vi "Main.vi"   [LabVIEW 2021]
uses:
  Hello World Event/Hello World Event/Hello World Event.lvclass
  C:/Program Files/National Instruments/LabVIEW 2021/vi.lib/Nathan Davis/jettl/jettl/Event/Event.lvclass
  <vilib>/Nathan Davis/jettl/jettl/jettl.lvlib
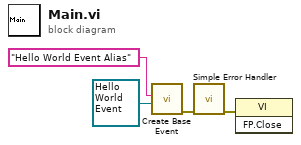
[diagram p0: block diagram]
diagram:
  n1 = call <vilib>:"Create Base Event.vi"("Event"=refnum<class "Hello World Event.lvclass"> refnum ("TEMPLATE Event.lvlib:TEMPLATE Event.lvclass"), "Self Event Alias"="Hello World Event Alias") -> ("error out"=w2:errorcluster)  [unwired: 9 in]
  n2 = call <vilib>:"Simple Error Handler.vi"("error in (no error)"=w2) -> ("error out"=w1:errorcluster)  [unwired: 4 in, 4 out]
  n3 = invoke class="VI" method="FP.Close"(error in=w1) -> ()  [unwired: 2 in, 3 out]
